vi "Observe.vi"(8 "error in (no error)":errorcluster, 10 "New Value":dbl, 11 "Histogram Ref":refnum<data-value>) -> (0 "error out":errorcluster, 3 "Histogram Ref out":refnum<data-value>)   [LabVIEW 2020, in "Metrics.lvlib" / "Histogram.lvclass"]
uses:
  Histogram.lvclass
  C:/Github-locals/PromVIEW/src/metrics/metric/Metric.lvclass
  Histogram.lvclass/Histogram.ctl
  metric/Metric.lvclass/Metric.ctl
  sample/Sample.lvclass/Sample.ctl
  sample/Read Value.vi
  sample/Write Value.vi
  Read Buckets.vi
  metric/Read Samples.vi
  metric/Write Samples.vi
  sample/Sample.lvclass
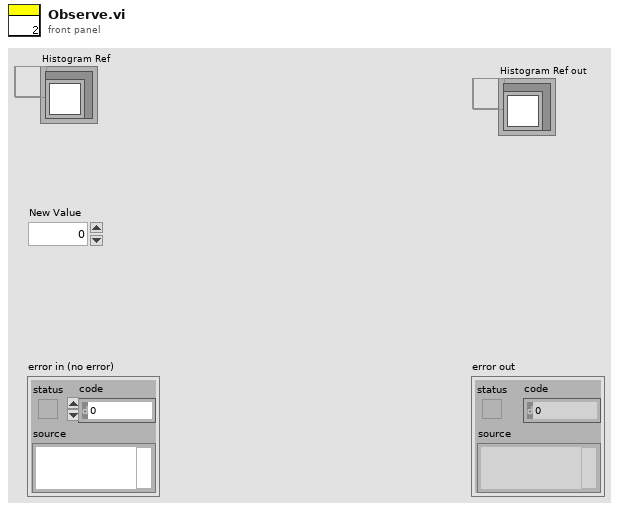
[diagram p1: front panel]
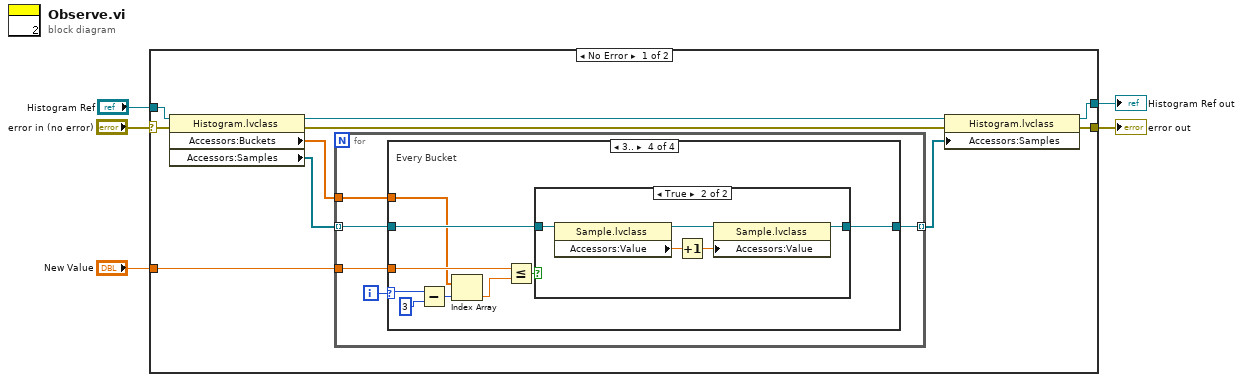
[diagram p0: block diagram]
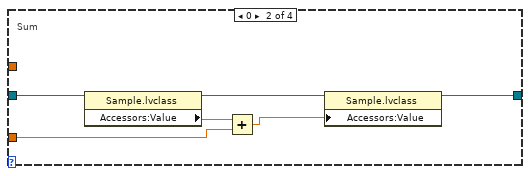
[diagram p3: hidden frame]
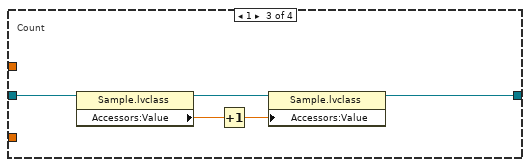
[diagram p4: hidden frame]
diagram:
  n1 = case shown="No Error" "error in (no error)" {
    selector: "error in (no error)" -> [w10 w49]
    tunnel: [w9 w49] -> w4
    tunnel: [w14 w48] -> w1
    tunnel: "Histogram Ref" -> [w15 w48]
    tunnel: "New Value" -> [w13 _]
    frame No Error {
      n2 = property class="Histogram.lvclass"(reference=w15, error in=w10) -> (reference out=w11:refnum<data-value>, error out=w8:errorcluster, "Accessors:Buckets"=w6:dbl[], "Accessors:Samples"=w7:refnum<class "Sample.lvclass">[])
      n3 = for {
        tunnel: w13 -> [w20]
        tunnel: w6 -> [w16]
        tunnel: w7 -> [w17] mode=indexing
        tunnel: [w18] -> w12 mode=indexing
        i -> [w19]
        n4 = case shown="3.." w19 {
          selector: w19 -> [_ _ _ w36]
          tunnel: w20 -> [_ w24 _ w40]
          tunnel: [w21 w23 w31 w41] -> w18
          tunnel: w17 -> [w21 w22 w28 w39]
          tunnel: w16 -> [_ _ _ w38]
          frame Default {
          }
          frame 0 {
            # "Sum"
            n5 = property class="Sample.lvclass"(reference=w22) -> (reference out=w27:refnum<class "Sample.lvclass">, "Accessors:Value"=w25:dbl)  [unwired: 1 in, 1 out]
            n6 = Add(x=w25, y=w24) -> (x+y=w26:dbl)
            n7 = property class="Sample.lvclass"(reference=w27, "Accessors:Value"=w26) -> (reference out=w23:refnum<class "Sample.lvclass">)  [unwired: 1 in, 1 out]
          }
          frame 1 {
            # "Count"
            n8 = property class="Sample.lvclass"(reference=w28) -> (reference out=w32:refnum<class "Sample.lvclass">, "Accessors:Value"=w30:dbl)  [unwired: 1 in, 1 out]
            n9 = Increment(x=w30) -> (x+1=w29:dbl)
            n10 = property class="Sample.lvclass"(reference=w32, "Accessors:Value"=w29) -> (reference out=w31:refnum<class "Sample.lvclass">)  [unwired: 1 in, 1 out]
          }
          frame 3.. {
            # "Every Bucket"
            n11 = Subtract(x=w36, y=3) -> (x-y=w37:i32)
            n12 = Index Array(array=w38, index=w37) -> (element=w33:dbl)
            n13 = Less Or Equal?(x=w40, y=w33) -> (x <= y?=w34:bool)
            n14 = case shown="True" w34 {
              tunnel: [w42 w46] -> w41
              tunnel: w39 -> [w42 w45]
              frame False {
              }
              frame True {
                n15 = property class="Sample.lvclass"(reference=w45) -> (reference out=w47:refnum<class "Sample.lvclass">, "Accessors:Value"=w44:dbl)  [unwired: 1 in, 1 out]
                n16 = Increment(x=w44) -> (x+1=w43:dbl)
                n17 = property class="Sample.lvclass"(reference=w47, "Accessors:Value"=w43) -> (reference out=w46:refnum<class "Sample.lvclass">)  [unwired: 1 in, 1 out]
              }
            }
          }
        }
      }
      n18 = property class="Histogram.lvclass"(reference=w11, error in=w8, "Accessors:Samples"=w12) -> (reference out=w14:refnum<data-value>, error out=w9:errorcluster)
    }
    frame Error {
    }
  }
  "error out" <- w4
  "Histogram Ref out" <- w1
